vi "물체를 만날시 회피하는 로봇.vi"() -> ()   [LabVIEW 2010]
uses:
  <vilib>/NXT/Block Support/NXT_InputPort.ctl
  <vilib>/NXT/Subs/MotorOutput.ctl
  <vilib>/NXT/Dual Mode Library/Waits/Wait_Num.vi
panel:
  in  "후진 시간":sgl=1.0
  in  "우 회전 시간":sgl=1.0
  in  "Power (75)":i32=75
  in  "Port (Port 4)":T1=3 items=["Port 1", "Port 2", "Port 3", "Port 4"]
  in  "stop":bool
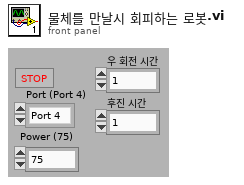
[diagram p1: front panel]
types:
  T1 = typedef "NXT_InputPort.ctl" = u8
  T2 = typedef "MotorOutput.ctl" = u8
  T3 = typedef "LVHSConnector.ctl" = cluster{"error":errorcluster, "address":string, "NXT #":i32, "Show Error":bool, "Connection":u16}
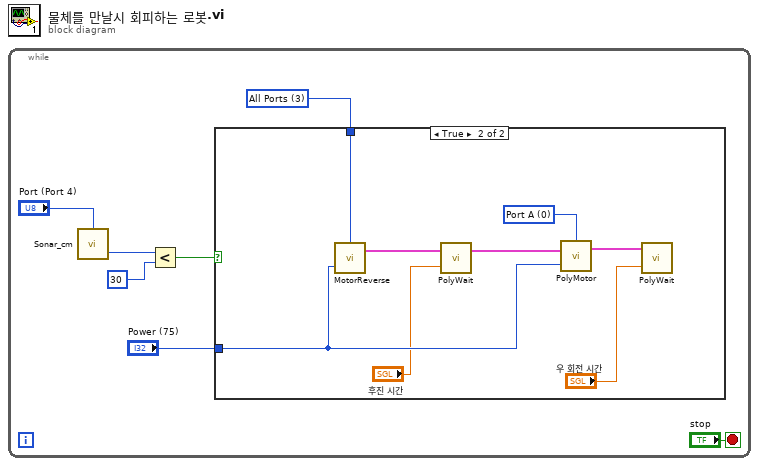
[diagram p0: block diagram]
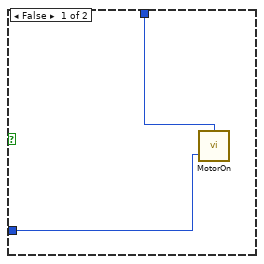
[diagram p2: hidden frame]
diagram:
  n1 = while {
    stop <- "stop" stop-if-true
    w1 = T2 3 items=["Port A", "Port B", "Port C", "All Ports"] ("Output Port (All Ports)")
    n2 = call <vilib>:"Sonar_cm.vi"("Port (Port 4)"="Port (Port 4)") -> ("Distance (cm)"=w4:i16)  [unwired: 2 in, 1 out]
    n3 = Less?(x=w4, y=i16 30) -> (x < y?=w5:bool)
    n4 = case shown="True" w5 {
      tunnel: "Power (75)" -> [w9 w13]
      tunnel: w1 -> [w8 w12]
      frame False {
        n5 = call <vilib>:"MotorOn.vi"("Power (75)"=w9, "Output Port (All Ports)"=w8) -> ()  [unwired: 2 in, 1 out]
      }
      frame True {
        w14 = T2 0 items=["Port A", "Port B", "Port C", "All Ports"] ("Output Port (All Ports)")
        n6 = call <vilib>:"MotorReverse.vi"("Power (75)"=w13, "Output Port (All Ports)"=w12) -> ("NXT"=w15:T3)  [unwired: 2 in]
        n7 = call-poly <vilib>:"PolyWait.vi"("Time (sec)"="후진 시간", "NXT"=w15) -> ("NXT"=w17:T3)  [unwired: 2 in]
        n8 = call-poly <vilib>:"PolyMotor.vi"("Power (75)"=w13, "NXT"=w17, "Output Port (All Ports)"=w14) -> ("NXT"=w16:T3)  [unwired: 1 in]
        n9 = call-poly <vilib>:"PolyWait.vi"("Time (sec)"="우 회전 시간", "NXT"=w16) -> ()  [unwired: 2 in, 1 out]
      }
    }
  }
